vi "ConnectWire.vi"(0 "__args":T1) -> (1 "__return":i32, 2 "__errStatus":bool, 3 "__errCode":i32, 4 "__errSource":string)   [LabVIEW 2013]
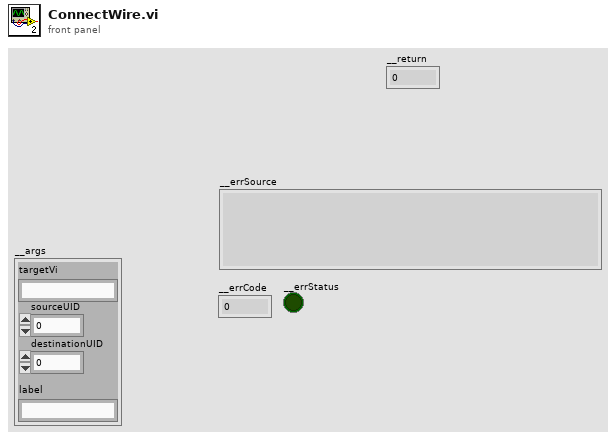
[diagram p1: front panel]
types:
  T1 = cluster{"targetVi":string, "sourceUID":i32, "destinationUID":i32, "label":string}
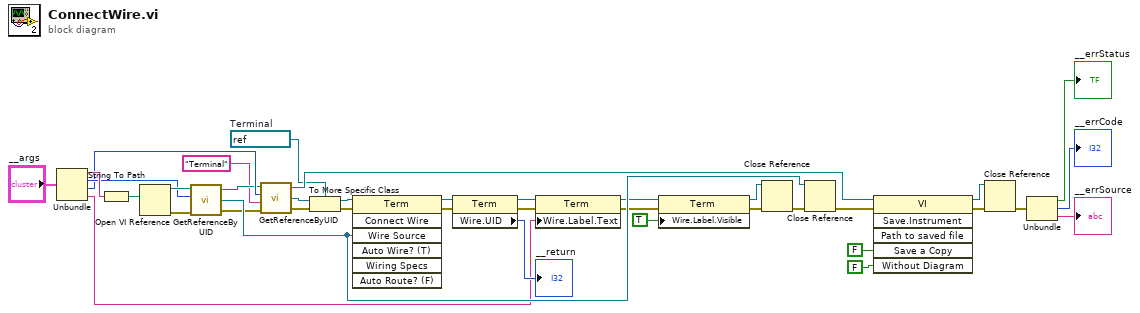
[diagram p0: block diagram]
diagram:
  w10 = refnum<vi> refnum  # Terminal
  n1 = Unbundle("__args") -> ("targetVi"=w27:string, "sourceUID"=w26:i32, "destinationUID"=w25:i32, "label"=w6:string)
  n2 = String To Path(string=w27) -> (path=w34:path)
  n3 = Open VI Reference(vi path=w34) -> (vi reference=w33:refnum<vi>, error out=w32:errorcluster)  [unwired: 5 in]
  n4 = call "GetReferenceByUID.vi"("error in (no error)"=w32, "UID"=w26, "targetVI"=w33) -> ("error out"=w12:errorcluster, "refNum"=w13:refnum<vi>, "dup targetVI"=w24:refnum<vi>)  [unwired: 1 in]
  n5 = call "GetReferenceByUID.vi"("error in (no error)"=w12, "objectClass"="Terminal", "UID"=w25, "targetVI"=w24) -> ("error out"=w22:errorcluster, "refNum"=w21:refnum<vi>, "dup targetVI"=w23:refnum<vi>)
  n6 = To More Specific Class(target class=w10, reference=w21, error in=w22) -> (specific class reference=w20:refnum<vi>, error out=w19:errorcluster)
  n7 = invoke class="Term" method="Connect Wire"(reference=w20, error in=w19, "Wire Source"=w13) -> (reference out=w16:refnum<vi>, error out=w14:errorcluster)  [unwired: 4 in, 5 out]
  n8 = property class="Term"(reference=w16, error in=w14) -> (reference out=w8:refnum<vi>, error out=w7:errorcluster, "Wire.UID"=→"__return":i32)
  n9 = property class="Term"(reference=w8, error in=w7, "Wire.Label.Text"=w6) -> (reference out=w2:refnum<vi>, error out=w5:errorcluster)
  n10 = property class="Term"(reference=w2, error in=w5, "Wire.Label.Visible"=TRUE ("Connected Wire.Label.Visible")) -> (reference out=w3:refnum<vi>, error out=w4:errorcluster)
  n11 = Close Reference(reference=w3, error in (no error)=w4) -> (error out=w17:errorcluster)
  n12 = Close Reference(reference=w13, error in (no error)=w17) -> (error out=w18:errorcluster)
  n13 = invoke class="VI" method="Save.Instrument"(reference=w23, error in=w18, "Save a Copy"=FALSE, "Without Diagram"=FALSE) -> (reference out=w31:refnum<vi>, error out=w30:errorcluster)  [unwired: 2 in, 4 out]
  n14 = Close Reference(reference=w31, error in (no error)=w30) -> (error out=w11:errorcluster)
  n15 = Unbundle(w11) -> ("status"=→"__errStatus":bool, "code"=→"__errCode":i32, "source"=→"__errSource":string)
